vi "Video still, with averaging.vi"(4 "Averaging time (s) (from end)":dbl=1.0, 5 "Interface name":T1="cam0", 6 "Duration (s)":dbl=4.0, 7 "VideoMode":u32, 8 "Image name":string="test", 9 "Image directory path":path=path "C:/test", 10 "FPS":u32=30, 11 "Video codec":string="Microsoft Video 1") -> (0 "Error Out":errorcluster, 3 "Image file path":path=path "C:/test/test.jpg")   [LabVIEW 2014]
doc: "Use this VI to acquire a time-averaged still frame. A temporary video stream of specified duration is acquired and frames over a specified duration from the end of the video are averaged together and output as a single frame. This VI will prove useful in obtaining cleaner snapshots from grainy footage, as well as bypassing the initial auto-exposure and auto-colour sequence of some webcams."
uses:
  <vilib>/userdefined/High Color/IMAQdx.ctl
  <vilib>/vision/driver/IMAQdx.llb/IMAQdx Camera Control Mode.ctl
  <vilib>/vision/driver/NI_Vision_Acquisition_Software.lvlib
  <resource>/objmgr/imaqdx.rc
  <vilib>/vision/NI_Vision_Development_Module.lvlib
panel:
  out "Image":T2(plugin-control)
  # "enter 0 for single end frame"
  # "PN 05/02/2015"
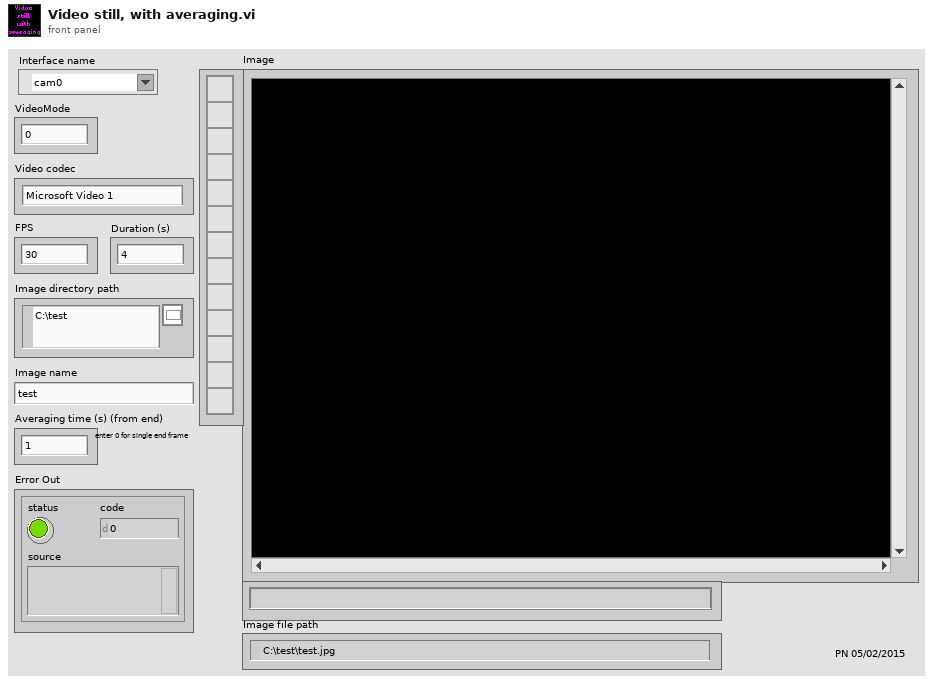
[diagram p1: front panel]
types:
  T1 = typedef "IMAQdx.ctl" = refnum<k21>
  T2 = typedef "IMAQ Image.ctl" = refnum<image>
  T3 = typedef "Image Type" = u32
  T4 = typedef "NI_Vision_Acquisition_Software.lvlib/IMAQdx Camera Control Mode.ctl" = enum32{"Controller", "Listener"}
  T5 = typedef "IMAQ AVI2 Refnum.ctl" = refnum<k20>
  T6 = cluster{"Width":u32, "Height":u32, "Frames Per Second":u32, "Codec":string, "Has Data":bool}
  T7 = cluster{"Red (or Hue) value":u8, "Green (or Sat) value":u8, "Blue (or Light or Val) value":u8}[][]
  T8 = cluster{"Red or Hue value":u8, "Green or Sat value":u8, "Blue or Luma or Val or Inten value":u8}
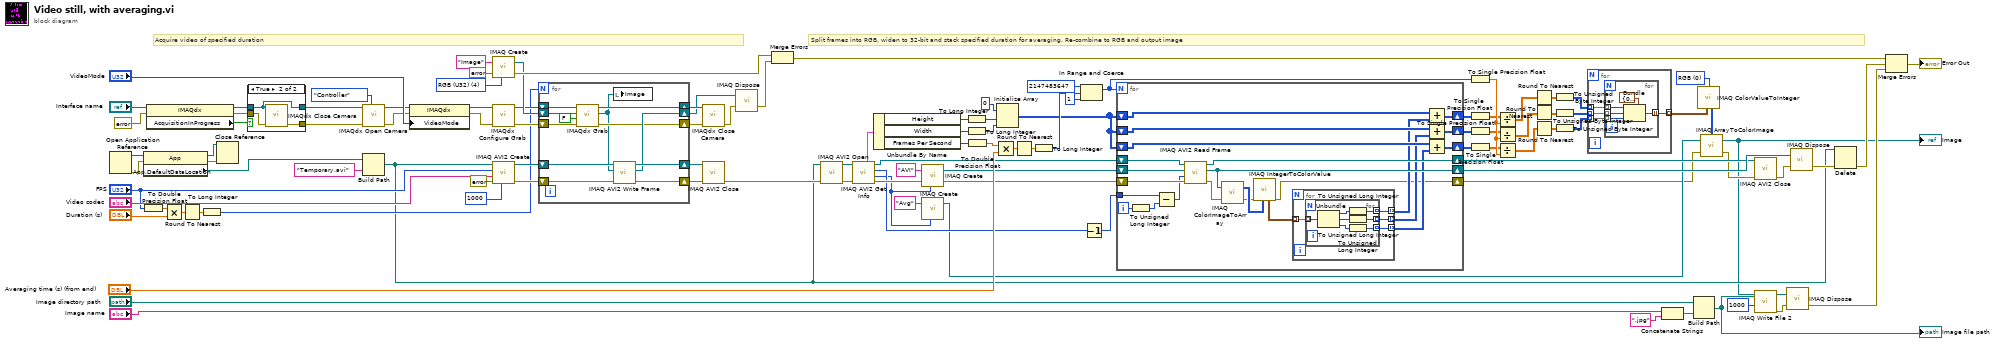
[diagram p0: block diagram]
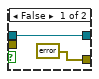
[diagram p2: hidden frame]
diagram:
  w26 = u16 0 items=["RGB", "HSL", "HSV", "HSI"] ("Color Mode")
  w108 = T3 4 items=["Grayscale (U8)", "Grayscale (I16)", "Grayscale (SGL)", "Complex (CSG)", "RGB (U32)", "HSL (U32)", "RGB (U64)", "Grayscale (U16)"] ("Image Type")
  # "Split frames into RGB, widen to 32-bit and stack specified duration for averaging. Re-combine to RGB and output image"
  # "Acquire video of specified duration"
  n1 = Open Application Reference() -> (0:w79:errorcluster, 3:w80:refnum<vi>)  [unwired: 4 in]
  n2 = To Double Precision Float(number="FPS") -> (double precision float=w2:dbl)
  n3 = property class="App"(reference=w80, error in=w79) -> (reference out=w77:refnum<vi>, error out=w76:errorcluster, "App.DefaultDataLocation"=w78:path)
  n4 = property class="IMAQdx"(reference="Interface name", error in=errorcluster {"status"=FALSE, "code"=0, "source"=""}) -> (reference out=w83:T1, error out=w85:errorcluster, "AcquisitionInProgress"=w84:bool)
  n5 = Multiply(x=w2, y="Duration (s)") -> (x*y=w73:dbl)
  n6 = Round To Nearest(number=w73) -> (nearest integer value=w1:dbl)
  n7 = To Long Integer(number=w1) -> (32bit integer=w72:i32)
  n8 = Close Reference(reference=w77, error in (no error)=w76) -> ()  [unwired: 1 out]
  n9 = case shown="True" w84 {
    tunnel: w83 -> [w114 w115]
    tunnel: w85 -> [_ w117]
    tunnel: [errorcluster {"status"=FALSE, "code"=0, "source"=""} ("error in") w116] -> w81
    tunnel: [w114 w115] -> w82
    frame False {
    }
    frame True {
      n10 = call <vilib>:"IMAQdx Close Camera.vi"("error in"=w117, "Session In"=w115) -> ("error out"=w116:errorcluster)  [unwired: 9 in]
    }
  }
  n11 = call <vilib>:"IMAQdx Open Camera.vi"("Camera Control Mode"=IMAQdx_Camera_Control_Mode."Controller", "error in"=w81, "Session In"=w82) -> ("error out"=w93:errorcluster, "Session Out"=w91:T1)  [unwired: 7 in]
  n12 = Build Path(base path=w78, name or relative path="Temporary.avi") -> (appended path=w48:path)
  n13 = property class="IMAQdx"(reference=w91, error in=w93, "VideoMode"="VideoMode") -> (reference out=w94:T1, error out=w92:errorcluster)
  n14 = call "IMAQ Create"("Image Name"="Image", "Image Type"=w108, "error in (no error)"=errorcluster {"status"=FALSE, "code"=0, "source"=""} ("error in")) -> ("New Image"=w106:T2, "error out"=w107:errorcluster)  [unwired: 2 in]
  n15 = call <vilib>:"IMAQdx Configure Grab.vi"("error in"=w92, "Session In"=w94) -> ("error out"=w103:errorcluster, "Session Out"=w95:T1)  [unwired: 8 in]
  n16 = call "IMAQ AVI2 Create"("Quality"=1000, "error in (no error)"=errorcluster {"status"=FALSE, "code"=0, "source"=""} ("error in"), "Codec"="Video codec", "Frames Per Second"="FPS", "AVI Path"=w48) -> ("error out"=w101:errorcluster, "AVI Refnum"=w102:T5)  [unwired: 5 in]
  n17 = for {
    N: w72 -> [_]
    shift-right: [w127] -> w105
    shift-left: w95 -> [w129]
    shift-right: [w121] -> w100
    shift-left: w106 -> [w128]
    shift-right: [w119] -> w104
    shift-left: w103 -> [w126]
    shift-right: [w123] -> w96
    shift-left: w102 -> [w124]
    shift-right: [w120] -> w97
    shift-left: w101 -> [w122]
    n18 = call <vilib>:"IMAQdx Grab.vi"("error in"=w126, "Wait for Next Buffer? (Yes)"=FALSE, "Image In"=w128, "Session In"=w129) -> ("error out"=w119:errorcluster, "Image Out"=w118:T2, "Session Out"=w127:T1)  [unwired: 4 in, 1 out]
    n19 = local write "Image"(w118) -> ()
    n20 = call "IMAQ AVI2 Write Frame"("error in (no error)"=w122, "Image"=w118, "AVI Refnum"=w124) -> ("error out"=w120:errorcluster, "Image Out (duplicate)"=w121:T2, "AVI Refnum (duplicate)"=w123:T5)  [unwired: 6 in]
  }
  n21 = call <vilib>:"IMAQdx Close Camera.vi"("error in"=w104, "Session In"=w105) -> ("error out"=w99:errorcluster)  [unwired: 9 in]
  n22 = call "IMAQ AVI2 Close"("error in (no error)"=w97, "AVI Refnum"=w96) -> ("error out"=w66:errorcluster)  [unwired: 9 in]
  n23 = call "IMAQ Dispose"("Image"=w100, "error in (no error)"=w99) -> ("error out"=w98:errorcluster)  [unwired: 4 in]
  n24 = Merge Errors(w107, w98) -> (w52:errorcluster)
  n25 = call "IMAQ AVI2 Open"("error in (no error)"=w66, "AVI File Path"=w48) -> ("error out"=w69:errorcluster, "AVI Refnum"=w68:T5)  [unwired: 8 in]
  n26 = call "IMAQ AVI2 Get Info"("error in (no error)"=w69, "AVI Refnum"=w68) -> ("error out"=w70:errorcluster, "Image Type"=w33:T3, "Number of Frames"=w35:u32, "AVI Refnum (duplicate)"=w59:T5, "Frame Data"=w31:T6)  [unwired: 5 in]
  n27 = Unbundle By Name(w31) -> ("Height"=w7:u32, "Width"=w6:u32, "Frames Per Second"=w63:u32)
  n28 = call "IMAQ Create"("Image Name"="AVI", "Image Type"=w33, "error in (no error)"=w70) -> ("New Image"=w41:T2, "error out"=w60:errorcluster)  [unwired: 2 in]
  n29 = call "IMAQ Create"("Image Name"="Avg", "Image Type"=w33) -> ("New Image"=w29:T2)  [unwired: 3 in, 1 out]
  n30 = To Long Integer(number=w7) -> (32bit integer=w5:i32)
  n31 = To Long Integer(number=w6) -> (32bit integer=w4:i32)
  n32 = To Double Precision Float(number=w63) -> (double precision float=w64:dbl)
  n33 = Multiply(x=w64, y="Averaging time (s) (from end)") -> (x*y=w62:dbl)
  n34 = Initialize Array(u32 0, w5, w4) -> (w30:u32[][])
  n35 = Round To Nearest(number=w62) -> (nearest integer value=w61:dbl)
  n36 = To Long Integer(number=w61) -> (32bit integer=w57:i32)
  n37 = In Range and Coerce(upper limit=2147483647, x=w57, lower limit=1) -> (coerced(x)=w34:i32)  [unwired: 1 out]
  n38 = Decrement(x=w35) -> (x-1=w36:u32)
  n39 = for {
    N: w34 -> [_]
    shift-right: [w130] -> w28
    shift-left: w60 -> [w152]
    shift-right: [w138] -> w54
    shift-left: w41 -> [w151]
    shift-right: [w149] -> w53
    shift-left: w59 -> [w150]
    tunnel: w36 -> [w148]
    shift-right: [w144] -> w14
    shift-left: w30 -> [w143]
    shift-right: [w142] -> w13
    shift-left: w30 -> [w139]
    shift-right: [w141] -> w12
    shift-left: w30 -> [w140]
    i -> [w147]
    n40 = To Unsigned Long Integer(number=w147) -> (unsigned 32bit integer=w145:u32)
    n41 = Subtract(x=w148, y=w145) -> (x-y=w146:u32)
    n42 = call "IMAQ AVI2 Read Frame"("error in (no error)"=w152, "Frame Number"=w146, "Image"=w151, "AVI Refnum"=w150) -> ("error out"=w132:errorcluster, "Image Out"=w138:T2, "AVI Refnum (duplicate)"=w149:T5)  [unwired: 5 in]
    n43 = call "IMAQ ColorImageToArray"("Image"=w138, "error in (no error)"=w132) -> ("Image Pixels (U32)"=w137:u32[][], "error out"=w131:errorcluster)  [unwired: 2 in, 1 out]
    n44 = call "IMAQ IntegerToColorValue"("error in (no error)"=w131, "2D U32 array"=w137) -> ("2D Color value array"=w136:T7, "error out"=w130:errorcluster)  [unwired: 3 in, 2 out]
    n45 = for {
      tunnel: w136 -> [w156] mode=indexing
      tunnel: [w155] -> w135 mode=indexing
      tunnel: [w154] -> w134 mode=indexing
      tunnel: [w153] -> w133 mode=indexing
      n46 = for {
        tunnel: w156 -> [w163] mode=indexing
        tunnel: [w159] -> w155 mode=indexing
        tunnel: [w158] -> w154 mode=indexing
        tunnel: [w157] -> w153 mode=indexing
        n47 = Unbundle(w163) -> ("Red (or Hue) value"=w162:u8, "Green (or Sat) value"=w160:u8, "Blue (or Light or Val) value"=w161:u8)
        n48 = To Unsigned Long Integer(number=w162) -> (unsigned 32bit integer=w159:u32)
        n49 = To Unsigned Long Integer(number=w160) -> (unsigned 32bit integer=w158:u32)
        n50 = To Unsigned Long Integer(number=w161) -> (unsigned 32bit integer=w157:u32)
      }
    }
    n51 = Add(x=w140, y=w135) -> (x+y=w141:u32[][])
    n52 = Add(x=w139, y=w134) -> (x+y=w142:u32[][])
    n53 = Add(x=w143, y=w133) -> (x+y=w144:u32[][])
  }
  n54 = To Single Precision Float(number=w34) -> (single precision float=w11:sgl)
  n55 = To Single Precision Float(number=w12) -> (single precision float=w10:sgl[][])
  n56 = To Single Precision Float(number=w13) -> (single precision float=w9:sgl[][])
  n57 = To Single Precision Float(number=w14) -> (single precision float=w8:sgl[][])
  n58 = Divide(x=w10, y=w11) -> (x/y=w25:sgl[][])
  n59 = Divide(x=w9, y=w11) -> (x/y=w24:sgl[][])
  n60 = Divide(x=w8, y=w11) -> (x/y=w23:sgl[][])
  n61 = Round To Nearest(number=w25) -> (nearest integer value=w22:sgl[][])
  n62 = Round To Nearest(number=w24) -> (nearest integer value=w21:sgl[][])
  n63 = Round To Nearest(number=w23) -> (nearest integer value=w20:sgl[][])
  n64 = To Unsigned Byte Integer(number=w22) -> (unsigned 8bit integer=w17:u8[][])
  n65 = To Unsigned Byte Integer(number=w21) -> (unsigned 8bit integer=w18:u8[][])
  n66 = To Unsigned Byte Integer(number=w20) -> (unsigned 8bit integer=w19:u8[][])
  n67 = for {
    tunnel: w19 -> [w167] mode=indexing
    tunnel: w18 -> [w166] mode=indexing
    tunnel: w17 -> [w165] mode=indexing
    tunnel: [w164] -> w16 mode=indexing
    n68 = for {
      tunnel: w167 -> [w171] mode=indexing
      tunnel: w166 -> [w170] mode=indexing
      tunnel: w165 -> [w169] mode=indexing
      tunnel: [w168] -> w164 mode=indexing
      n69 = Bundle(cluster=T8 {"Red or Hue value"=0, "Green or Sat value"=0, "Blue or Luma or Val or Inten value"=0} ("Color Value"), "Red or Hue value"=w169, "Green or Sat value"=w170, "Blue or Luma or Val or Inten value"=w171) -> (w168:T8)
    }
  }
  n70 = Concatenate Strings("Image name", ".jpg" ("name or relative path")) -> (w46:string)
  n71 = Build Path(base path="Image directory path", name or relative path=w46) -> (appended path=w47:path)
  "Image file path" <- w47
  n72 = call "IMAQ ColorValueToInteger"("2D Color value array"=w16, "Color Mode"=w26) -> ("2D U32 array"=w15:u32[][])  [unwired: 3 in, 3 out]
  n73 = call "IMAQ ArrayToColorImage"("Image Pixels (U32)"=w15, "Image"=w29, "error in (no error)"=w28) -> ("Image Out"=w3:T2, "error out"=w27:errorcluster)  [unwired: 2 in]
  "Image" <- w3
  n74 = call "IMAQ AVI2 Close"("error in (no error)"=w27, "AVI Refnum"=w53) -> ("error out"=w55:errorcluster)  [unwired: 9 in]
  n75 = call-poly "IMAQ Write File 2"("Image Quality"=u32 1000, "File Path"=w47, "Image"=w3) -> ("error out"=w44:errorcluster, "Image Out (duplicate)"=w43:T2)  [unwired: 7 in]
  n76 = call "IMAQ Dispose"("Image"=w43, "error in (no error)"=w44) -> ("error out"=w37:errorcluster)  [unwired: 4 in]
  n77 = call "IMAQ Dispose"("Image"=w54, "error in (no error)"=w55) -> ("error out"=w51:errorcluster)  [unwired: 4 in]
  n78 = Delete(path (use dialog)=w48, error in=w51) -> (error out=w50:errorcluster)  [unwired: 3 in, 2 out]
  n79 = Merge Errors(w52, w50, w37) -> (→"Error Out":errorcluster)
